vi "Construct.vi"(8 "error in (no error)":errorcluster, 9 "Default Language":string="en") -> (0 "error out":errorcluster, 3 "LangFile out":refnum<class "Resource Data.lvclass">)   [LabVIEW 2013, in "SET Project Data.lvlib" / "Resource Data.lvclass"]
uses:
  Resource Data.lvclass
  Resource Data.lvclass/Resource Data.ctl
  SET Project Data.lvlib
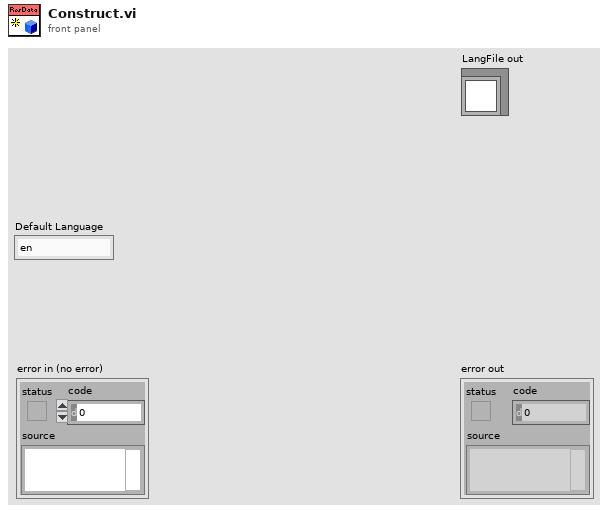
[diagram p1: front panel]
types:
  T1 = typedef "SET Project Data.lvlib/ProjFile_Language Entry.ctl" = cluster{"Tag":string, "Name":string, "Code Page":u16}
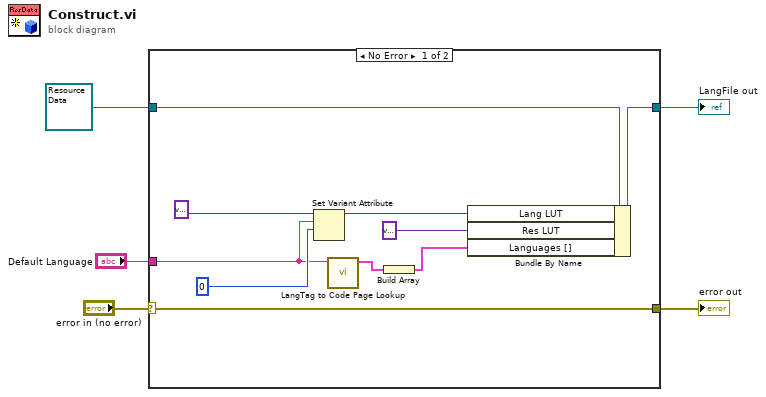
[diagram p0: block diagram]
diagram:
  n1 = case shown="No Error" "error in (no error)" {
    selector: "error in (no error)" -> [w14 w17]
    tunnel: [w14 w17] -> w4
    tunnel: refnum<class "Resource Data.lvclass"> refnum ("LangFile in") -> [w13 w16]
    tunnel: "Default Language" -> [w9 _]
    tunnel: [w15 w16] -> w1
    frame No Error {
      n2 = Set Variant Attribute(Variant=variant ("RID LUT"), name=w9, value=0) -> (Variant out=w10:variant)  [unwired: 1 in, 2 out]
      n3 = call "LangTag to Code Page Lookup.vi"("Tag"=w9) -> ("Language"=w7:T1)  [unwired: 9 in, 1 out]
      n4 = Build Array(w7) -> (w8:T1[])
      n5 = Bundle By Name(cluster=w13, "Lang LUT"=w10, "Res LUT"=variant ("RID LUT"), "Languages []"=w8) -> (w15:refnum<class "Resource Data.lvclass">)
    }
    frame Error {
    }
  }
  "error out" <- w4
  "LangFile out" <- w1
